vi "Get Server Key File.vi"(11 "OOP Server in":refnum<class "HVC3.lvclass">) -> (2 "Server Key File (.key)":path, 3 "OOP Server out":refnum<class "HVC3.lvclass">)   [LabVIEW 2019, in "HVC3.lvlib" / "HVC3.lvclass"]
uses:
  HVC3.lvclass
  HVC3.lvclass/HVC3.ctl
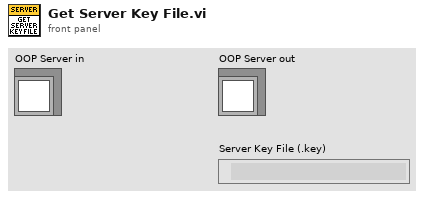
[diagram p1: front panel]
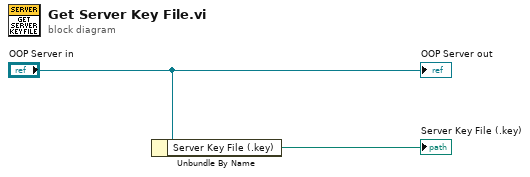
[diagram p0: block diagram]
diagram:
  n1 = Unbundle By Name("OOP Server in") -> ("Server Key File (.key)"=→"Server Key File (.key)":path)
  "OOP Server out" <- "OOP Server in"
